vi "BaseName.vi"(1 "Path":path) -> (0 "Name":string)   [LabVIEW 2014]
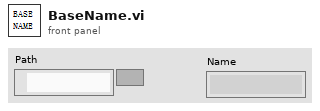
[diagram p1: front panel]
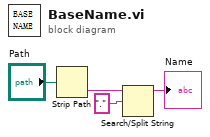
[diagram p0: block diagram]
diagram:
  n1 = Strip Path(path="Path") -> (name=w3:string)  [unwired: 1 out]
  n2 = Search/Split String(string=w3, search string/char (-)=".") -> (substring before match=→"Name":string)  [unwired: 1 in, 2 out]
